vi "XY Graph Add Multiplots with Names.vi"(0 "XYGraph in":T3, 1 "Array of Scales (Default)":cluster{"X Scale":u32, "Y Scale":u32}[](array[cluster]), 2 "Plots Interpolation (Previous Plot's Style)":T2[](array[typedef]) items=["Point (.)", "Stepwise Right (--.)", "Line + Point (\\. /)", "Stepwise Left (.--)", "Stepwise Centered (-.-)", "Stepwise Vertical (|.|)", "Line (-)", "Use Previous Plot's Style"], 3 "Keep Existing Plots (T)":bool=TRUE, 5 "Array of Plots":cluster{"X Array":dbl[], "Y Array":dbl[]}[](array[cluster]), 7 "Plots Metadata":variant[](array[variant]), 9 "Array of Plot Names (\"Plot\")":string[](array[string]), 11 "error in (no error)":errorcluster, 12 "Make Visible (T)":bool=TRUE, 13 "Plot Colors (Default)":u32[](array[colorbox]), 14 "Point Style (Dot)":T1=enum."Dot") -> (4 "XY Graph Caption":string, 6 "Total Number of Plots":i32, 8 "Number of Plots Added":i32, 10 "Added Plot Names":string[](array[string]), 15 "error out":errorcluster)   [LabVIEW 2019]
uses:
  XY Graph Refnum.ctl
  LabVIEW Plot Interpolation.ctl
  Plot Point Style.ctl
  XY Graph Add-Ons.lvlib
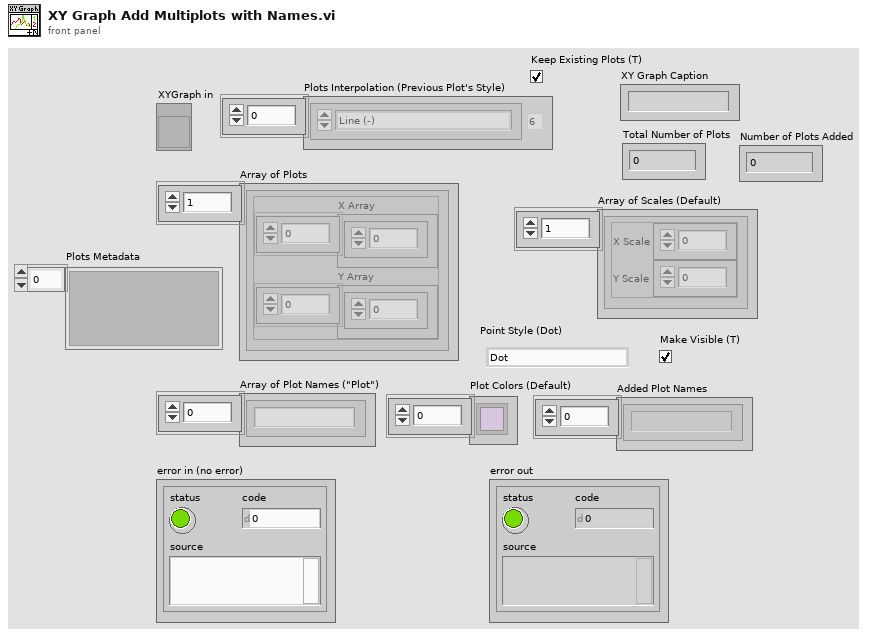
[diagram p1: front panel]
types:
  T1 = typedef "Plot Point Style.ctl" = enum16{"not defined", "None", "Empty Circle", "Filled Circle", "Thick Circle", "Dotted Circle", "Empty Square", "Filled Square", "Thick Square", "Dotted Square", "Small Filled Square", "Dot", "Cross", "Tiny Cross", "Large X", "Small x", "Diamond", "Small Empty Square"}
  T2 = typedef "LabVIEW Plot Interpolation.ctl" = u8
  T3 = typedef "XY Graph Add-Ons.lvlib/XY Graph Refnum.ctl" = refnum<vi>
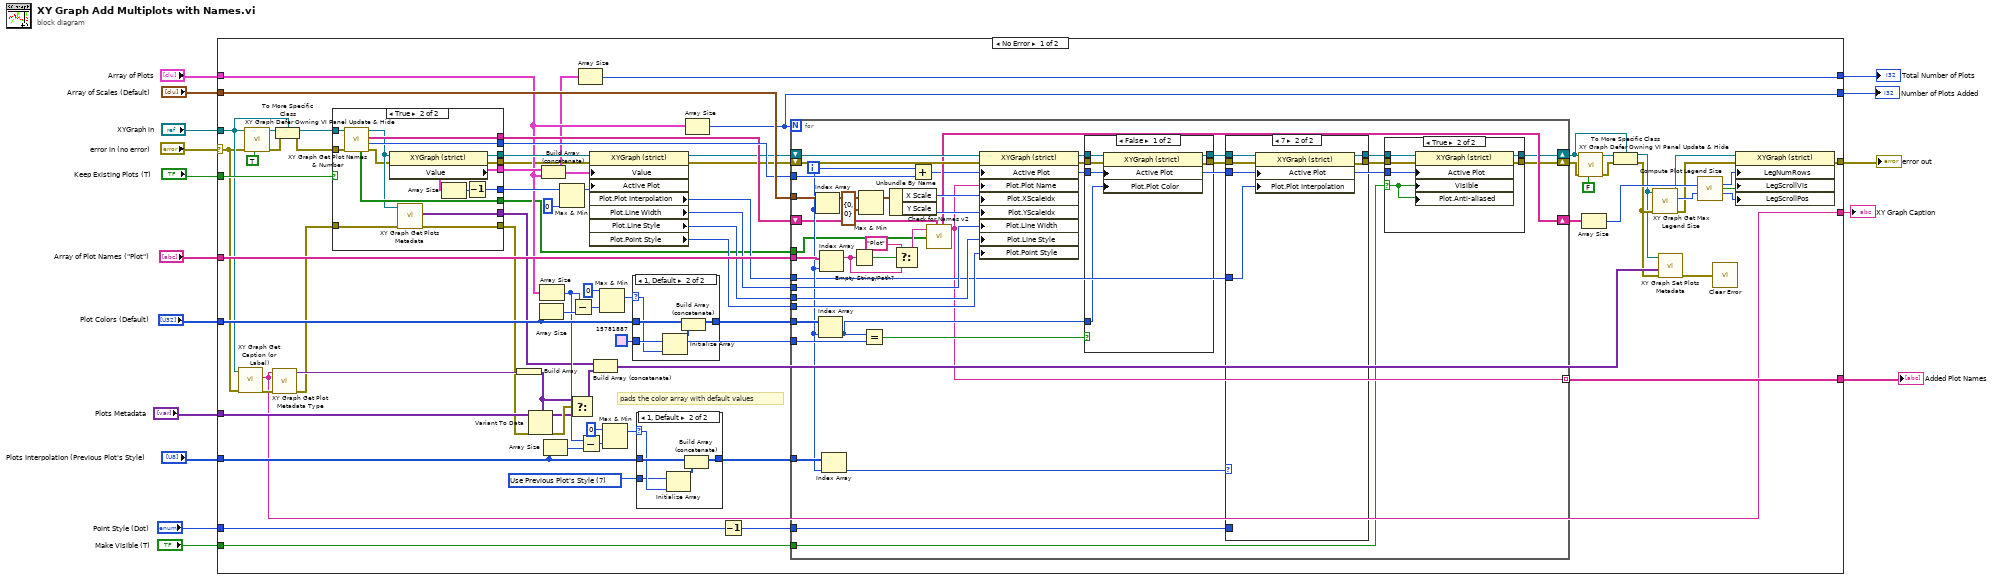
[diagram p0: block diagram]
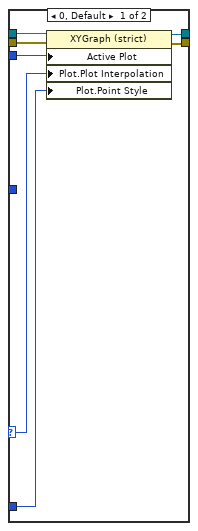
[diagram p3: hidden frame]
diagram:
  n1 = case shown="No Error" "error in (no error)" {
    selector: "error in (no error)" -> [w19 w193]
    tunnel: "XYGraph in" -> [w29 _]
    tunnel: "Array of Plot Names (\"Plot\")" -> [w91 _]
    tunnel: "Array of Scales (Default)" -> [w90 _]
    tunnel: [w81 _] -> w12
    tunnel: "Array of Plots" -> [w80 _]
    tunnel: "Plot Colors (Default)" -> [w76 _]
    tunnel: "Plots Interpolation (Previous Plot's Style)" -> [w73 _]
    tunnel: "Keep Existing Plots (T)" -> [w62 _]
    tunnel: [w61 w193] -> w7
    tunnel: [w59 _] -> w6
    tunnel: "Point Style (Dot)" -> [w58 _]
    tunnel: "Make Visible (T)" -> [w56 _]
    tunnel: [w54 _] -> w3
    tunnel: [w17 _] -> w2
    tunnel: "Plots Metadata" -> [w27 _]
    frame No Error {
      w66 = T2 7 items=["Point (.)", "Stepwise Right (--.)", "Line + Point (\\. /)", "Stepwise Left (.--)", "Stepwise Centered (-.-)", "Stepwise Vertical (|.|)", "Line (-)", "Use Previous Plot's Style"] ("Plot Interpolation")
      w74 = u32 15781887 ("Plot Color (Default)")
      # "pads the color array with default values"
      n2 = call "XY Graph Get Caption (or Label).vi"("error in (no error)"=w19, "XYGraph in"=w29) -> ("error out"=w18:errorcluster, "Caption (or Label) Text"=w17:string)  [unwired: 7 in, 1 out]
      n3 = call "XY Graph Defer Owning VI Panel Update & Hide.vi"("Defer Owning Panel Update"=TRUE, "error in (no error)"=w19, "XY Graph Refnum in"=w29) -> ("error out"=w45:errorcluster, "XY Graph Refnum out"=w48:refnum<vi>)  [unwired: 7 in]
      n4 = call "XY Graph Get Plot Metadata Type.vi"("Error In"=w18, "Graph Label"=w17) -> ("Error Out"=w22:errorcluster, "Plot Metadata Type"=w28:variant)  [unwired: 7 in, 1 out]
      n5 = To More Specific Class(target class=w29, reference=w48, error in=w45) -> (specific class reference=w46:T3, error out=w44:errorcluster)
      n6 = case shown="True" w62 {
        tunnel: [w165 w180] -> w92
        tunnel: w46 -> [w165 w179]
        tunnel: w44 -> [w164 w178]
        tunnel: [_ w177] -> w89
        tunnel: [_ w175] -> w88
        tunnel: [_ w174] -> w87
        tunnel: [_ w173] -> w86
        tunnel: [w164 w172] -> w55
        tunnel: [_ w171] -> w47
        tunnel: [_ w169] -> w33
        tunnel: w22 -> [w163 w167]
        tunnel: [w163 w166] -> w21
        frame False {
        }
        frame True {
          n7 = call "XY Graph Get Plot Names & Number.vi"("error in (no error)"=w178, "XYGraph in"=w179) -> ("error out"=w168:errorcluster, "# Plots"=w174:i32, "Plot Names"=w173:string[], "XYGraph out"=w170:T3, "Empty Plots?"=w171:bool[])  [unwired: 5 in]
          n8 = property class="XYGraph (strict)"(reference=w170, error in=w168) -> (reference out=w180:T3, error out=w172:errorcluster, "Value"=w177:cluster{"X Array":dbl[], "Y Array":dbl[]}[])
          n9 = call "XY Graph Get Plots Metadata.vi"("Error In"=w167, "XYGraph Ref"=w170) -> ("Error Out"=w166:errorcluster, "Plots Metadata"=w169:variant[])  [unwired: 6 in, 2 out]
          n10 = Array Size(array=w177) -> (size(s)=w176:i32)
          n11 = Decrement(x=w176) -> (x-1=w175:i32)
        }
      }
      n12 = Build Array(w28) -> (w24:variant[])
      n13 = Variant To Data(error in=w21, type=w24, Variant=w27) -> (data=w25:variant[], error out=w26:errorcluster)
      n14 = Array Size(array=w76) -> (size(s)=w71:i32)
      n15 = Array Size(array=w80) -> (size(s)=w65:i32)
      n16 = Build Array (concatenate)(w89, w80) -> (w60:cluster{"X Array":dbl[], "Y Array":dbl[]}[])
      n17 = Array Size(array=w73) -> (size(s)=w72:i32)
      n18 = Max & Min(x=w88, y=0) -> (max(x,y)=w64:i32)  [unwired: 1 out]
      n19 = Select(t=w24, s=w26, f=w25) -> (s? t:f=w23:variant[])
      n20 = Subtract(x=w65, y=w71) -> (x-y=w79:i32)
      n21 = Array Size(array=w60) -> (size(s)=w59:i32)
      n22 = Subtract(x=w65, y=w72) -> (x-y=w70:i32)
      n23 = property class="XYGraph (strict)"(reference=w92, error in=w55, "Value"=w60, "Active Plot"=w64) -> (reference out=w53:T3, error out=w52:errorcluster, "Plot.Plot Interpolation"=w85:u8, "Plot.Line Width"=w84:u8, "Plot.Line Style"=w83:u8, "Plot.Point Style"=w82:u8)
      n24 = Build Array (concatenate)(w33, w23) -> (w32:variant[])
      n25 = Max & Min(x=0, y=w79) -> (max(x,y)=w77:i32)  [unwired: 1 out]
      n26 = Max & Min(x=0, y=w70) -> (max(x,y)=w68:i32)  [unwired: 1 out]
      n27 = case shown="1, Default" w77 {
        selector: w77 -> [_ w190]
        tunnel: w76 -> [w187 w192]
        tunnel: [w187 w191] -> w75
        tunnel: w74 -> [_ w188]
        frame 0 {
        }
        frame 1, Default {
          n28 = Initialize Array(w188, w190) -> (w189:u32[])
          n29 = Build Array (concatenate)(w192, w189) -> (w191:u32[])
        }
      }
      n30 = case shown="1, Default" w68 {
        selector: w68 -> [_ w184]
        tunnel: w73 -> [w181 w186]
        tunnel: [w181 w185] -> w67
        tunnel: w66 -> [_ w182]
        frame 0 {
        }
        frame 1, Default {
          n31 = Initialize Array(w182, w184) -> (w183:T2[])
          n32 = Build Array (concatenate)(w186, w183) -> (w185:T2[])
        }
      }
      n33 = Array Size(array=w80) -> (size(s)=w54:i32)
      n34 = Decrement(x=w58) -> (x-1=w57:T1)
      n35 = for {
        N: w54 -> [_]
        tunnel: w91 -> [w130]
        shift-right: [w98] -> w51
        shift-left: w52 -> [w132]
        shift-right: [w101] -> w36
        shift-left: w53 -> [w133]
        tunnel: w87 -> [w131]
        shift-right: [w104] -> w93
        shift-left: w86 -> [w105]
        tunnel: w90 -> [w129]
        tunnel: w85 -> [w107]
        tunnel: w84 -> [w122]
        tunnel: w83 -> [w121]
        tunnel: w82 -> [w120]
        tunnel: [w102] -> w81 mode=indexing
        tunnel: w75 -> [w119]
        tunnel: w74 -> [w118]
        tunnel: w67 -> [w110]
        tunnel: w57 -> [w106]
        tunnel: w56 -> [w100]
        tunnel: w47 -> [w94]
        i -> [w109]
        n36 = Index Array(array=w129, index=w109) -> (element=w128:cluster{"X Scale":u32, "Y Scale":u32})
        n37 = Index Array(array=w119, index=w109) -> (element=w114:u32)
        n38 = Index Array(array=w130, index=w109) -> (element=w124:string)
        n39 = Index Array(array=w110, index=w109) -> (element=w108:T2)
        n40 = Empty String/Path?(string/path=w124) -> (empty?=w125:bool)
        n41 = Max & Min(x=w128, y=cluster{"X Scale":u32, "Y Scale":u32} {"X Scale"=0, "Y Scale"=0}) -> (max(x,y)=w96:cluster{"X Scale":u32, "Y Scale":u32})  [unwired: 1 out]
        n42 = Equal?(x=w114, y=w118) -> (x = y?=w117:bool)
        n43 = Unbundle By Name(w96) -> ("X Scale"=w127:u32, "Y Scale"=w126:u32)
        n44 = Select(t="Plot", s=w125, f=w124) -> (s? t:f=w103:string)
        n45 = Add(x=w109, y=w131) -> (x+y=w97:i32)
        n46 = call "Check for Names v2.vi"("New Name"=w103, "Name List"=w105, "Empty Plots?"=w94) -> ("New Name List"=w104:string[], "New Name"=w102:string)  [unwired: 3 in, 2 out]
        n47 = property class="XYGraph (strict)"(reference=w133, error in=w132, "Active Plot"=w97, "Plot.Plot Name"=w102, "Plot.XScaleIdx"=w127, "Plot.YScaleIdx"=w126, "Plot.Line Width"=w122, "Plot.Line Style"=w121, "Plot.Point Style"=w120) -> (reference out=w116:T3, error out=w115:errorcluster)
        n48 = case shown="False" w117 {
          tunnel: w116 -> [w160 w162]
          tunnel: [w159 w162] -> w113
          tunnel: w115 -> [w158 w161]
          tunnel: [w157 w161] -> w112
          tunnel: w114 -> [w156 _]
          tunnel: w97 -> [w155 _]
          frame False {
            n49 = property class="XYGraph (strict)"(reference=w160, error in=w158, "Active Plot"=w155, "Plot.Plot Color"=w156) -> (reference out=w159:T3, error out=w157:errorcluster)
          }
          frame True {
          }
        }
        n50 = case shown="7" w108 {
          selector: w108 -> [w143 _]
          tunnel: w113 -> [w148 w154]
          tunnel: [w147 w153] -> w111
          tunnel: w112 -> [w146 w152]
          tunnel: [w145 w151] -> w99
          tunnel: w97 -> [w144 w150]
          tunnel: w107 -> [_ w149]
          tunnel: w106 -> [w142 _]
          frame 0, Default {
            n51 = property class="XYGraph (strict)"(reference=w148, error in=w146, "Active Plot"=w144, "Plot.Plot Interpolation"=w143, "Plot.Point Style"=w142) -> (reference out=w147:T3, error out=w145:errorcluster)
          }
          frame 7 {
            n52 = property class="XYGraph (strict)"(reference=w154, error in=w152, "Active Plot"=w150, "Plot.Plot Interpolation"=w149) -> (reference out=w153:T3, error out=w151:errorcluster)
          }
        }
        n53 = case shown="True" w100 {
          selector: w100 -> [_ w136]
          tunnel: w111 -> [w135 w141]
          tunnel: [w135 w140] -> w101
          tunnel: w99 -> [w134 w139]
          tunnel: [w134 w138] -> w98
          tunnel: w97 -> [_ w137]
          frame False {
          }
          frame True {
            n54 = property class="XYGraph (strict)"(reference=w141, error in=w139, "Active Plot"=w137, "Visible"=w136, "Plot.Anti-aliased"=w136) -> (reference out=w140:T3, error out=w138:errorcluster)
          }
        }
      }
      n55 = call "XY Graph Defer Owning VI Panel Update & Hide.vi"("Defer Owning Panel Update"=FALSE, "error in (no error)"=w51, "XY Graph Refnum in"=w36) -> ("error out"=w38:errorcluster, "XY Graph Refnum out"=w37:refnum<vi>)  [unwired: 7 in]
      n56 = Array Size(array=w93) -> (size(s)=w42:i32)
      n57 = To More Specific Class(target class=w36, reference=w37, error in=w38) -> (specific class reference=w30:T3, error out=w31:errorcluster)
      n58 = call "XY Graph Get Max Legend Size.vi"("Error In"=w31, "XYGraph Refnum"=w30) -> ("Error Out"=w34:errorcluster, "Max Legend Size"=w43:i32, "XYGraph Refnum"=w35:T3)  [unwired: 6 in, 1 out]
      n59 = call "XY Graph Set Plots Metadata.vi"("error in (no error)"=w31, "Plots Metadata"=w32, "XY Graph Refnum"=w30) -> ("error out"=w20:errorcluster)  [unwired: 7 in, 1 out]
      n60 = call "Compute Plot Legend Size.vi"("# Plots"=w42, "Max Legend Size"=w43) -> ("LegNumRows"=w41:u32, "LegScrollVis"=w40:bool, "LegScrollPos"=w39:u32)  [unwired: 11 in]
      n61 = call "Clear Error.vi"("Error In"=w20) -> ()  [unwired: 8 in, 1 out]
      n62 = property class="XYGraph (strict)"(reference=w35, error in=w34, "LegNumRows"=w41, "LegScrollVis"=w40, "LegScrollPos"=w39) -> (error out=w61:errorcluster)  [unwired: 1 out]
    }
    frame Error {
    }
  }
  "error out" <- w7
  "Added Plot Names" <- w12
  "Total Number of Plots" <- w6
  "Number of Plots Added" <- w3
  "XY Graph Caption" <- w2
